vi "Array Max & Min String.vi"(7 "JSON Array":refnum<class "JSON Helper.lvclass">, 11 "error in (no error)":errorcluster) -> (4 "max value":refnum<class "JSON String.lvclass">, 6 "max index":i32, 8 "min value":refnum<class "JSON String.lvclass">, 10 "min index":i32, 15 "error out":errorcluster)   [LabVIEW 2016]
uses:
  JSON Helper/JSON Helper.lvclass
  JSON Helper/To More Specific Type (String).vi
  JSON Datatype/JSON Null.lvclass
  JSON String/JSON String.lvclass
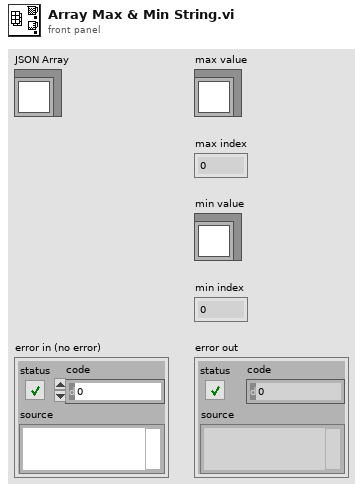
[diagram p1: front panel]
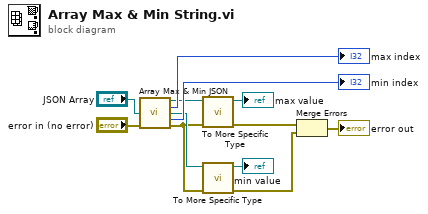
[diagram p0: block diagram]
diagram:
  n1 = call "Array Max & Min JSON.vi"("JSON Array"="JSON Array", "error in (no error)"="error in (no error)") -> ("max value"=w8:refnum<class "JSON Helper.lvclass">, "max index"=→"max index":i32, "min value"=w7:refnum<class "JSON Helper.lvclass">, "min index"=→"min index":i32, "error out"=w6:errorcluster)  [unwired: 9 in]
  n2 = call-poly "To More Specific Type.vi"("error in (no error)"=w6, "JSON Datatype in"=w8) -> ("error out"=w3:errorcluster, "JSON Datatype out"=→"max value":refnum<class "JSON String.lvclass">)  [unwired: 8 in]
  n3 = call-poly "To More Specific Type.vi"("error in (no error)"=w6, "JSON Datatype in"=w7) -> ("error out"=w4:errorcluster, "JSON Datatype out"=→"min value":refnum<class "JSON String.lvclass">)  [unwired: 8 in]
  n4 = Merge Errors(w3, w4) -> (→"error out":errorcluster)
